vi "Vision Processing.vi"(8 "error in (no error)":errorcluster, 11 "Image Size":T1=enum."320x240") -> ()   [LabVIEW 2016]
uses:
  Vision Support Code/Camera Types.ctl
  <vilib>/Rock Robotics/WPI/Camera/WPI_CameraImageSize.ctl
  <vilib>/Rock Robotics/WPI/Camera/WPI_CameraWhite Balance Values.ctl
  <vilib>/Rock Robotics/WPI/Camera/WPI_CameraExposure Values.ctl
  <vilib>/Rock Robotics/WPI/Camera/WPI_CameraFrameRate.ctl
  Robot Global Data.vi
  <vilib>/Rock Robotics/Network Tables/NT Write Number.vi
  <vilib>/vision/NI_Vision_Development_Module.lvlib
panel:
  out "loop ms":u32
  out "Calibration error":errorcluster
  in  "Display Original":bool
  in  "Display Mask":bool
  in  "Line Border":cluster{"Top":dbl, "Bottom":dbl}={"Top"=6.0, "Bottom"=1.0}
  in  "Use Calibration":bool=TRUE
  out "Instructions:":string="Use Source to load image files from a directory, or use a USB or IP camera connected to your laptop. Use Camera Settings 1 and 2 to achieve a dark image with bright and colorful stripes.\nLED Color can encoded as HSL or related color modes. Calibrate to the same color as the strips being reflected to the camera.\nClick and draw a line in Original Image to auto-calibrate the LED Color. You may want to widen and tweak Sat and Val by hand.\nThe Annotate button affects drawing a rectangle around the stripes and labeling it with a distance in ft. Distance relies on knowing the Camera Type and lens calibration (it looks up the lens view angle).\n\nAdjust Score Cutoff to make the code more or less picky. If the color is not very unique, you may need to increase the number of particles considered. The diagram uses a Size Limit to ignore colored things that are too small. You may need to adjust it if you are targetting from far away.\n\nResults give you the distance to the target, the center and box in a normalized (-1 to 1) and pixel coordinates.\n\nBe sure to read about setting camera exposure and brightness to help simplify your image and acquire color saturated images.\n\nThere are lots of comments on the diagram to explain the code."
  in  "Color Mode":u16(ring)=3 items=["RGB", "HSL", "HSV", "HSI"]
  in  "Particles":dbl=5.0
  in  "Score Cutoff %":dbl=70.0
  in  "Camera Type":T2=enum."MS HD3000 square"
  out "Results":T3 {"Score" format="%#_3g"; "Pixels"."Rectangle"."Numeric 5" format="%#_3g"; "Pixels"."Rectangle"."Numeric 3" format="%#_3g"; "Pixels"."Rectangle"."Numeric 2" format="%#_3g"; "Pixels"."Rectangle"."Numeric" format="%#_3g"; "Normalized"."Rectangle"."Numeric 5" format="%#_2g"; "Normalized"."Rectangle"."Numeric 3" format="%#_2g"; "Normalized"."Rectangle"."Numeric 2" format="%#_2g"; "Normalized"."Rectangle"."Numeric" format="%#_2g"; "Normalized"."Center"."?" format="%#_3g"; "Normalized"."Center"."?" format="%#_3g"; "Distance (ft)" format="%#_3g"}
  out "Qualified Particles":i32
  in  "LED Color":T4={"Hue"={107.81818389892578, 139.81818389892578}, "Sat"={176.07142857142858, 255.0}, "Val"={40.53571428571429, 255.0}} {"Hue" scale=0.0..255.0 scale format="%#_3g"}
  out "Mask":T5(plugin-control)
  out "Original Image":T5(plugin-control)
  # "Legend:\n    Rectangle\n       Green - Good target, distance ft\n       Red - Bad target\n    Orange Text - Score in %"
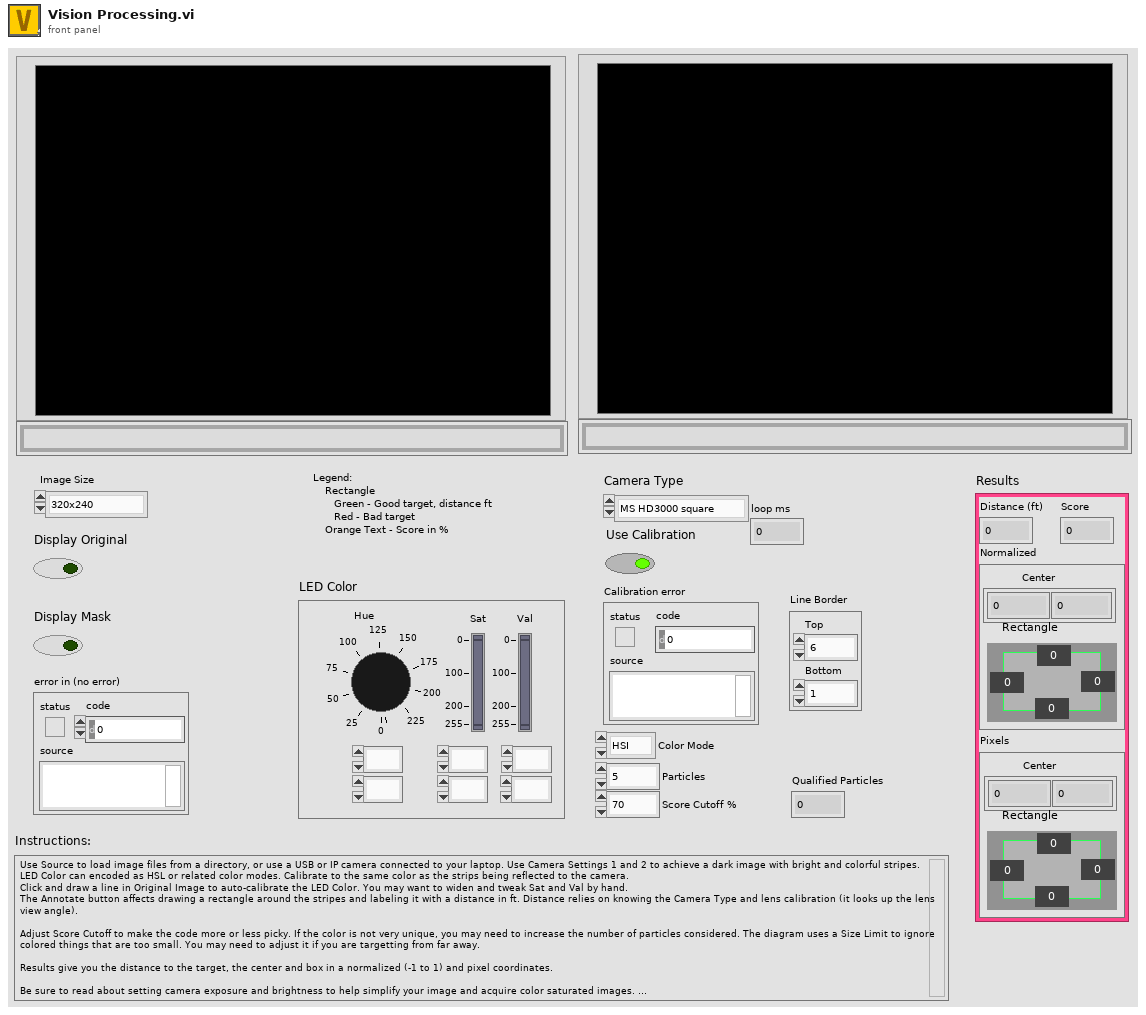
[diagram p1: front panel]
types:
  T1 = typedef "WPI_CameraImageSize.ctl" = enum16{"640x480", "320x240", "160x120", "Custom"}
  T2 = typedef "Camera Types.ctl" = enum16{"206", "1011", "1013", "MS HD3000 square", "MS HD3000 640x480"}
  T3 = cluster{"Distance (ft)":dbl, "Score":dbl, "Normalized":cluster{"Center":cluster{dbl, dbl}, "Rectangle":cluster{"Numeric":dbl, "Numeric 2":dbl, "Numeric 3":dbl, "Numeric 5":dbl}}, "Pixels":cluster{"Center":cluster{dbl, dbl}, "Rectangle":cluster{"Numeric":dbl, "Numeric 2":dbl, "Numeric 3":dbl, "Numeric 5":dbl}}}
  T4 = cluster{"Hue":cluster{dbl, dbl}, "Sat":cluster{dbl, dbl}, "Val":cluster{dbl, dbl}}
  T5 = typedef "IMAQ Image.ctl" = refnum<image>
  T6 = typedef "WPI_CameraFrameRate.ctl" = u32
  T7 = typedef "WPI_CameraExposure Values.ctl" = enum16{"Auto", "Flicker-free 50 Hz", "Flicker-free 60 Hz", "Hold current", "Custom"}
  T8 = typedef "WPI_CameraWhite Balance Values.ctl" = enum16{"Auto", "Fixed indoor", "Fixed outdoor 1", "Fixed outdoor 2", "Fixed fluorescent 1", "Fixed fluorescent 2", "Hold current", "Custom"}
  T9 = typedef "Image Type" = u32
  T10 = typedef "Particle Parameters" = i32
  T11 = typedef "WPI_CameraDevRef.ctl" = cluster{"Camera Address":string, "CameraStatus":errorcluster}
  T12 = cluster{"Left":dbl, "Top":dbl, "Right":dbl, "Bottom":dbl}
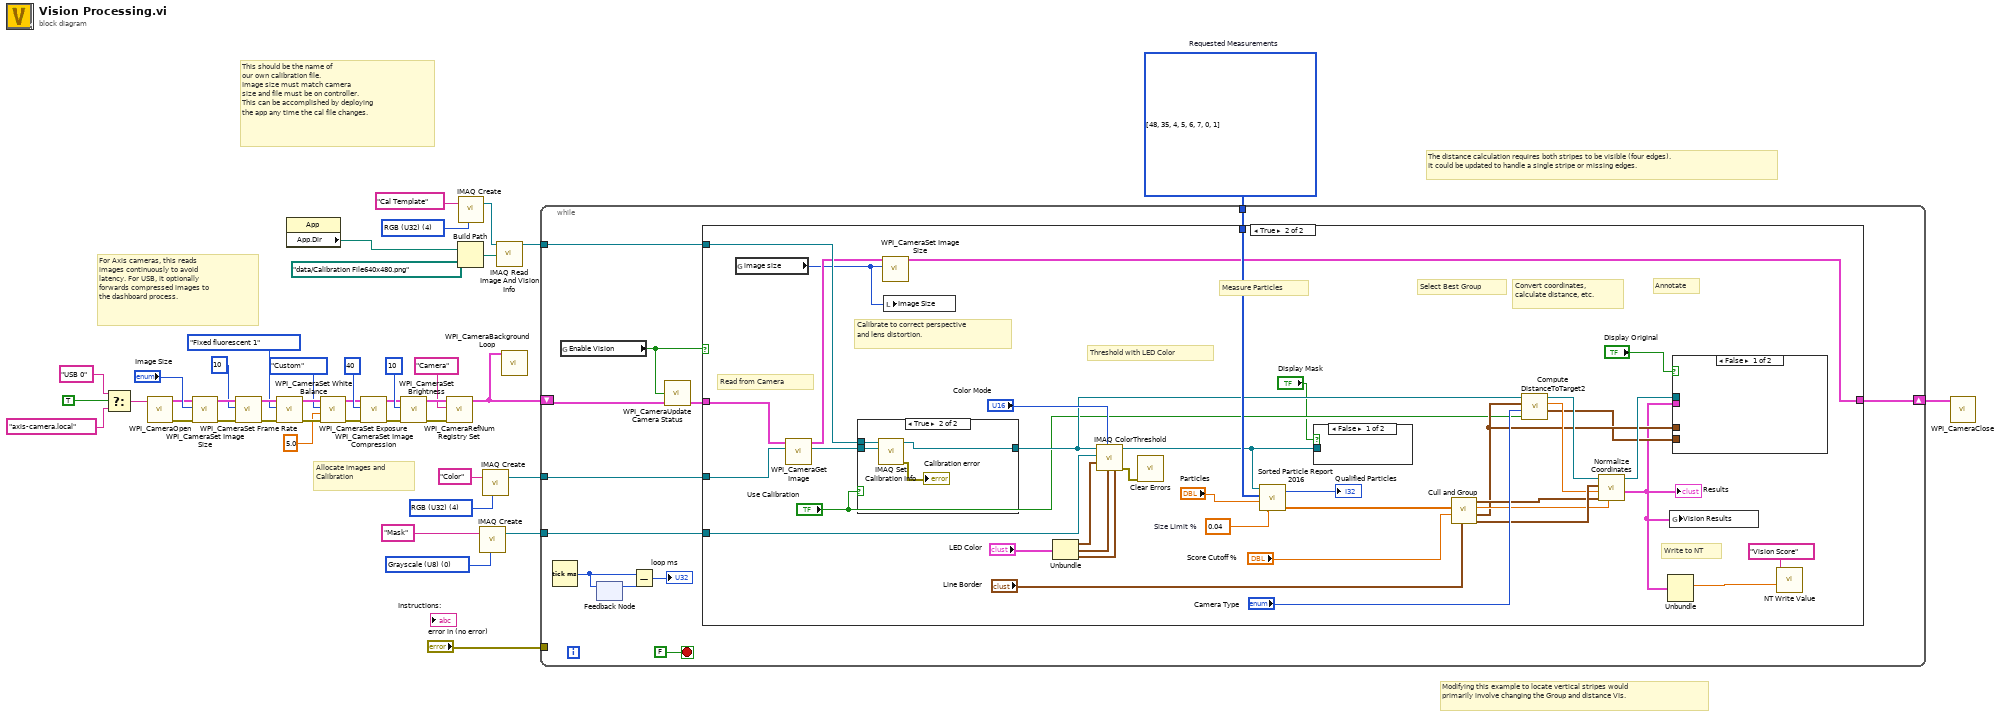
[diagram p0: block diagram]
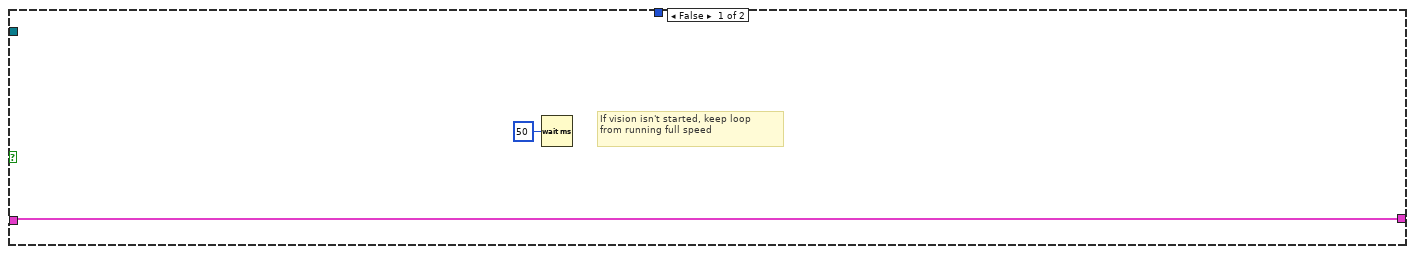
[diagram p2: hidden frame]
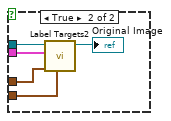
[diagram p3: hidden frame]
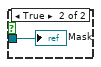
[diagram p4: hidden frame]
diagram:
  w36 = T9 4 items=["Grayscale (U8)", "Grayscale (I16)", "Grayscale (SGL)", "Complex (CSG)", "RGB (U32)", "HSL (U32)", "RGB (U64)", "Grayscale (U16)"] ("Image Type")
  w38 = T10[] [48, 35, 4, 5, 6, 7, 0, 1] items=["Center of Mass X", "Center of Mass Y", "First Pixel X", "First Pixel Y", "Bounding Rect Left", "Bounding Rect Top", "Bounding Rect Right", "Bounding Rect Bottom", "Max Feret Diameter Start X", "Max Feret Diameter Start Y", "Max Feret Diameter End X", "Max Feret Diameter End Y", "Max Horiz. Segment Length Left", "Max Horiz. Segment Length Right", "Max Horiz. Segment Length Row", "-", "Bounding Rect Width", "Bounding Rect Height", "Bounding Rect Diagonal", "Perimeter", "Convex Hull Perimeter", "Holes' Perimeter", "Max Feret Diameter", "Equivalent Ellipse Major Axis", "Equivalent Ellipse Minor Axis", "Equivalent Ellipse Minor Axis (Feret)", "Equivalent Rect Long Side", "Equivalent Rect Short Side", "Equivalent Rect Diagonal", "Equivalent Rect Short Side (Feret)", "Average Horiz. Segment Length", "Average Vert. Segment Length", "Hydraulic Radius", "Waddel Disk Diameter", "-", "Area", "Holes' Area", "Particle & Holes' Area", "Convex Hull Area", "Image Area", "-", "Number of Holes", "Number of Horiz. Segments", "Number of Vert. Segments", "-", "Orientation", "Max Feret Diameter Orientation", "-", "% Area/Image Area", "% Area/(Particle & Holes' Area)", "Ratio of Equivalent Ellipse Axes", "Ratio of Equivalent Rect Sides", "-", "Elongation Factor", "Compactness Factor", "Heywood Circularity Factor", "Type Factor", "-", "Sum X", "Sum Y", "Sum XX", "Sum XY", "Sum YY", "Sum XXX", "Sum XXY", "Sum XYY", "Sum YYY", "-", "Moment of Inertia XX", "Moment of Inertia XY", "Moment of Inertia YY", "Moment of Inertia XXX", "Moment of Inertia XXY", "Moment of Inertia XYY", "Moment of Inertia YYY", "Norm. Moment of Inertia XX", "Norm. Moment of Inertia XY", "Norm. Moment of Inertia YY", "Norm. Moment of Inertia XXX", "Norm. Moment of Inertia XXY", "Norm. Moment of Inertia XYY", "Norm. Moment of Inertia YYY", "Hu Moment 1", "Hu Moment 2", "Hu Moment 3", "Hu Moment 4", "Hu Moment 5", "Hu Moment 6", "Hu Moment 7"]  # Requested Measurements
  w41 = T9 0 items=["Grayscale (U8)", "Grayscale (I16)", "Grayscale (SGL)", "Complex (CSG)", "RGB (U32)", "HSL (U32)", "RGB (U64)", "Grayscale (U16)"] ("Image Type")
  w42 = T9 4 items=["Grayscale (U8)", "Grayscale (I16)", "Grayscale (SGL)", "Complex (CSG)", "RGB (U32)", "HSL (U32)", "RGB (U64)", "Grayscale (U16)"] ("Image Type")
  # "This should be the name of \nour own calibration file.\nImage size must match camera\nsize and file must be on controller.\nThis can be accomplished by deploying\nthe app any time the cal file changes."
  # "For Axis cameras, this reads\nimages continuously to avoid\nlatency. For USB, it optionally\nforwards compressed images to\nthe dashboard process."
  # "Modifying this example to locate vertical stripes would\nprimarily involve changing the Group and distance VIs."
  # "The distance calculation requires both stripes to be visible (four edges).\nIt could be updated to handle a single stripe or missing edges."
  # "Allocate images and\nCalibration"
  n1 = Select(t="USB 0" ("format string"), s=TRUE ("dot notation? (F)"), f="axis-camera.local" ("format string")) -> (s? t:f=w6:string)
  n2 = call <vilib>:"WPI_CameraOpen.vi"("Camera Address"=w6) -> ("error out"=w18:errorcluster, "CameraDevRef"=w19:T11)  [unwired: 1 in, 8 out]
  n3 = call <vilib>:"WPI_CameraSet Image Size.vi"("error in (no error)"=w18, "Image Size"="Image Size", "CameraDevRef"=w19) -> ("error out"=w17:errorcluster, "CameraDevRef Out"=w20:T11)  [unwired: 1 in, 6 out]
  n4 = call <vilib>:"WPI_CameraSet Frame Rate.vi"("error in (no error)"=w17, "Frame Rate (fps)"=T6 10, "CameraDevRef"=w20) -> ("error out"=w16:errorcluster, "CameraDevRef Out"=w22:T11)  [unwired: 7 out]
  n5 = call <vilib>:"WPI_CameraSet White Balance.vi"("error in (no error)"=w16, "White Balance"=WPI_CameraWhite_Balance_Values."Fixed fluorescent 1", "CameraDevRef"=w22) -> ("error out"=w15:errorcluster, "CameraDevRef Out"=w21:T11)  [unwired: 1 in, 6 out]
  n6 = property class="App"() -> ("App.Dir"=w1:path)  [unwired: 2 in, 2 out]
  n7 = call <vilib>:"WPI_CameraSet Exposure.vi"("error in (no error)"=w15, "Exposure (%)"=5.0, "Exposure"=WPI_CameraExposure_Values."Custom", "CameraDevRef"=w21) -> ("error out"=w14:errorcluster, "CameraDevRef Out"=w24:T11)  [unwired: 6 out]
  n8 = call <vilib>:"WPI_CameraSet Image Compression.vi"("error in (no error)"=w14, "Compression"=40, "CameraDevRef"=w24) -> ("error out"=w13:errorcluster, "CameraDevRef Out"=w23:T11)  [unwired: 7 out]
  n9 = call <vilib>:"WPI_CameraSet Brightness.vi"("error in (no error)"=w13, "Brightness"=10, "CameraDevRef"=w23) -> ("error out"=w12:errorcluster, "CameraDevRef Out"=w30:T11)  [unwired: 7 out]
  n10 = call <vilib>:"WPI_CameraRefNum Registry Set.vi"("error in (no error)"=w12, "refnum name"="Camera", "CameraDevRef"=w30) -> ("CameraDevRef"=w5:T11)  [unwired: 1 in, 7 out]
  n11 = Build Path(base path=w1, name or relative path=path "data/Calibration File640x480.png" ("Folder Location")) -> (appended path=w32:path)
  n12 = call "IMAQ Create"("Image Name"="Cal Template", "Image Type"=w36) -> ("New Image"=w34:T5)  [unwired: 2 in, 2 out]
  n13 = call "IMAQ Create"("Image Name"="Mask", "Image Type"=w41) -> ("New Image"=w39:T5)  [unwired: 2 in, 2 out]
  n14 = call "IMAQ Create"("Image Name"="Color", "Image Type"=w42) -> ("New Image"=w37:T5)  [unwired: 2 in, 2 out]
  n15 = call "IMAQ Read Image And Vision Info"("File Path"=w32, "Image"=w34) -> ("Image Out"=w33:T5)  [unwired: 7 in, 2 out]
  n16 = call <vilib>:"WPI_CameraBackground Loop.vi"("CameraDevRef"=w5) -> ()  [unwired: 11 in]
  n17 = while {
    tunnel: w37 -> [w51]
    tunnel: w39 -> [w54]
    tunnel: w38 -> [w53]
    tunnel: w33 -> [w52]
    shift-right: [w50] -> w4
    shift-left: w5 -> [w49]
    tunnel: "error in (no error)" -> [_]
    stop <- FALSE stop-if-true
    n18 = Tick Count (ms)() -> (millisecond timer value=w45:u32)
    n19 = global read "Robot Global Data.vi" "Enable Vision"() -> (w47:bool)
    n20 = feedback-in #1(w45) -> ()
    n21 = feedback #1() -> (w46:u32)  [unwired: 1 in]
    n22 = Subtract(x=w45, y=w46) -> (x-y=→"loop ms":u32)
    n23 = call <vilib>:"WPI_CameraUpdate Camera Status.vi"("CameraDevRef In"=w49, "Enable Vision"=w47) -> ("CameraDevRef Out"=w48:T11)  [unwired: 3 in]
    n24 = case shown="True" w47 {
      tunnel: w54 -> [_ w95]
      tunnel: w53 -> [_ w91]
      tunnel: w52 -> [_ w71]
      tunnel: w48 -> [w57 w68]
      tunnel: w51 -> [_ w67]
      tunnel: [w57 w62] -> w50
      frame False {
        # "If vision isn't started, keep loop\nfrom running full speed"
        n25 = Wait (ms)(milliseconds to wait=u32 50) -> ()  [unwired: 1 out]
      }
      frame True {
        w89 = 0.04  # Size Limit %
        # "Write to NT"
        # "Read from Camera"
        # "Calibrate to correct perspective\nand lens distortion."
        # "Measure Particles"
        # "Convert coordinates,\ncalculate distance, etc."
        # "Annotate"
        # "Select Best Group"
        # "Threshold with LED Color"
        n26 = global read "Robot Global Data.vi" "image size"() -> (w61:T1)
        n27 = call <vilib>:"WPI_CameraGet Image.vi"("Image"=w67, "CameraDevRef"=w68) -> ("Image Out"=w66:T5, "CameraDevRef Out"=w63:T11)  [unwired: 7 in, 1 out]
        n28 = case shown="True" "Use Calibration" {
          tunnel: [w102 w106] -> w72
          tunnel: w66 -> [w102 w105]
          tunnel: w71 -> [_ w104]
          frame False {
          }
          frame True {
            n29 = call "IMAQ Set Calibration Info"("Image Dst"=w105, "Image Src"=w104) -> ("error out"=→"Calibration error":errorcluster, "Calibrated Image"=w106:T5)  [unwired: 8 in]
          }
        }
        n30 = call <vilib>:"WPI_CameraSet Image Size.vi"("Image Size"=w61, "CameraDevRef"=w63) -> ("CameraDevRef Out"=w62:T11)  [unwired: 2 in, 7 out]
        n31 = local write "Image Size"(w61) -> ()
        n32 = Unbundle("LED Color") -> ("Hue"=w94:cluster{dbl, dbl}, "Sat"=w93:cluster{dbl, dbl}, "Val"=w92:cluster{dbl, dbl})
        n33 = call "IMAQ ColorThreshold"("Blue or Luma or Val or Inten Range"=w92, "Green or Sat Range"=w93, "Color Mode"="Color Mode", "Red or Hue Range"=w94, "Image Dst"=w95, "Image Src"=w72) -> ("error out"=w88:errorcluster, "Image Dst Out"=w84:T5)  [unwired: 4 in]
        n34 = call <vilib>:"Clear Errors.vi"("error in (no error)"=w88) -> ()  [unwired: 5 in, 2 out]
        n35 = call "Sorted Particle Report 2016.vi"("Min Area Size %"=w89, "Particle Count Limit"="Particles", "Pixel Measurements"=w91, "Image in"=w84) -> ("Sorted Data"=w86:dbl[][], "Particles"=→"Qualified Particles":i32)
        n36 = case shown="False" "Display Mask" {
          tunnel: w84 -> [_ w101]
          frame False {
          }
          frame True {
            "Mask" <- w101
          }
        }
        n37 = call "Cull and Group.vi"("Line Border"="Line Border", "Score Cutoff"="Score Cutoff %", "Sorted Data"=w86) -> ("Rect"=w82:T12, "Line"=w74:T12, "Score"=w77:dbl, "Center"=w78:cluster{"X":dbl, "Y":dbl})  [unwired: 5 in]
        n38 = call "Compute DistanceToTarget2.vi"("Calibrated"="Use Calibration", "Camera Type"="Camera Type", "Line"=w74, "Image Src"=w72) -> ("Edges"=w73:cluster{"X":sgl, "Y":sgl}[], "Distance (ft)"=w81:dbl, "Image Dst Out"=w80:T5)  [unwired: 5 in]
        n39 = call "Normalize Coordinates.vi"("Score"=w77, "Center"=w78, "Distance"=w81, "Bounding box"=w82, "Image in"=w80) -> ("Results"=w60:T3, "Image out"=w79:T5)  [unwired: 5 in]
        "Results" <- w60
        n40 = Unbundle(w60) -> ("Score"=w59:dbl)  [unwired: 3 out]
        n41 = global write "Robot Global Data.vi" "Vision Results"(w60) -> ()
        n42 = case shown="False" "Display Original" {
          tunnel: w79 -> [_ w99]
          tunnel: w60 -> [_ w98]
          tunnel: w74 -> [_ w97]
          tunnel: w73 -> [_ w96]
          frame False {
          }
          frame True {
            n43 = call "Label Targets2.vi"("Edges"=w96, "Line"=w97, "Results"=w98, "Image in"=w99) -> ("Image out"=→"Original Image":T5)  [unwired: 7 in]
          }
        }
        n44 = call-poly <vilib>:"NT Write Value.vi"("Numeric"=w59, "Name"="Vision Score") -> ()  [unwired: 9 in, 1 out]
      }
    }
  }
  n45 = call <vilib>:"WPI_CameraClose.vi"("CameraDevRef"=w4) -> ()  [unwired: 1 in, 10 out]
